vi "get file data.vi"(8 "error in":errorcluster, 11 "Path":path) -> (0 "error out":errorcluster, 2 "format":T1)   [LabVIEW 2023, in "CEF.lvlib"]
doc: "Reads a full file and interprets it using <b>base file format.ctl</b>, which is a tuple of version and data.Copyright 2017 National Instruments Corporation\n\nLicensed under the Apache License, Version 2.0 (the \"License\"); you may not use this file except in compliance with the License. You may obtain a copy of the License at http://www.apache.org/licenses/LICENSE-2.0\nUnless required by applicable law or agreed to in writing, software distributed under the License is distributed on an \"AS IS\" BASIS, WITHOUT WARRANTIES OR CONDITIONS OF ANY KIND, either express or implied. See the License for the specific language governing permissions and limitations under the License."
uses:
  CEF.lvlib
  base file format.ctl
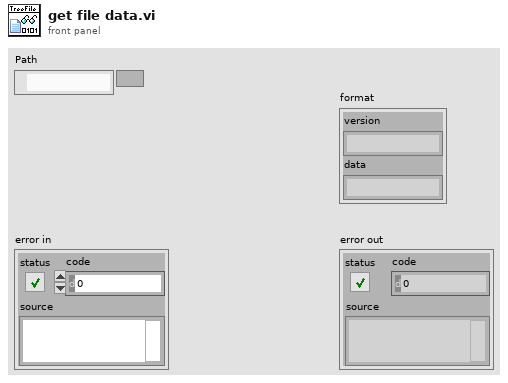
[diagram p1: front panel]
types:
  T1 = typedef "CEF.lvlib/base file format.ctl" = cluster{"version":string, "data":string}
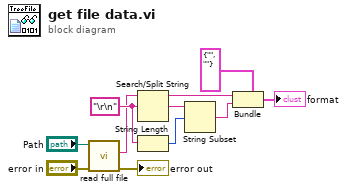
[diagram p0: block diagram]
diagram:
  w5 = "\r\n" ("String")
  n1 = call "read full file.vi"("error in"="error in", "file path"="Path") -> ("error out"=→"error out":errorcluster, "data"=w2:string)  [unwired: 8 in]
  n2 = Search/Split String(string=w2, search string/char (-)=w5) -> (substring before match=w9:string, match + rest of string=w7:string)  [unwired: 1 in, 1 out]
  n3 = String Length(string=w5) -> (length=w8:i32)
  n4 = String Subset(string=w7, offset (0)=w8) -> (substring=w6:string)  [unwired: 1 in]
  n5 = Bundle(cluster=T1 {"version"="", "data"=""} ("format"), "version"=w9, "data"=w6) -> (→"format":T1)
